vi "dfd_Check Project in Memory.vi"(8 "error in (no error)":errorcluster, 9 "filter name":string, 10 "dest path":path) -> (0 "error out":errorcluster, 1 "filter name out":string, 2 "dup dest path":path)   [LabVIEW 2017, in "NI_DigFilterLicensed.lvlib"]
uses:
  <vilib>/addons/Digital Filter Design/NI_DigFilterLicensed.lvlib
  <vilib>/addons/Digital Filter Design/_Misc.llb/dfd_Error Handlers (Single).vi
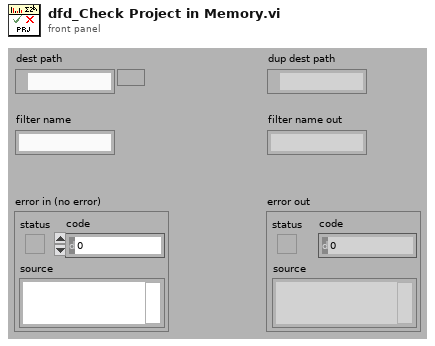
[diagram p1: front panel]
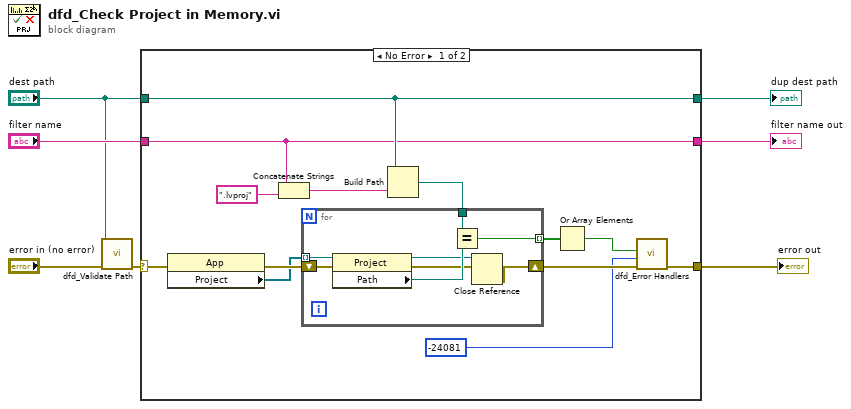
[diagram p0: block diagram]
diagram:
  n1 = call <vilib>:"dfd_Validate Path.vi"("error in (no error)"="error in (no error)", "path in"="dest path") -> ("error out"=w2:errorcluster)  [unwired: 9 out]
  n2 = case shown="No Error" w2 {
    selector: w2 -> [w18 w29]
    tunnel: "filter name" -> [w8 _]
    tunnel: "dest path" -> [w19 w30]
    tunnel: [w19 w30] -> w6
    tunnel: [w8 _] -> w5
    tunnel: [w9 w29] -> w4
    frame No Error {
      n3 = property class="App"(error in=w18) -> (error out=w13:errorcluster, "Project"=w12:refnum<vi>[])  [unwired: 1 in, 1 out]
      n4 = Concatenate Strings(w8, ".lvproj" ("string")) -> (w16:string)
      n5 = Build Path(base path=w19, name or relative path=w16) -> (appended path=w17:path)
      n6 = for {
        tunnel: w12 -> [w28] mode=indexing
        shift-right: [w21] -> w14
        shift-left: w13 -> [w27]
        tunnel: w17 -> [w25]
        tunnel: [w24] -> w15 mode=indexing
        n7 = property class="Project"(reference=w28, error in=w27) -> (reference out=w23:refnum<vi>, error out=w22:errorcluster, "Path"=w26:path)
        n8 = Equal?(x=w25, y=w26) -> (x = y?=w24:bool)
        n9 = Close Reference(reference=w23, error in (no error)=w22) -> (error out=w21:errorcluster)
      }
      n10 = Or Array Elements(Boolean array=w15) -> (logical OR=w11:bool)
      n11 = call-poly <vilib>:"dfd_Error Handlers.vi"("error in (no error)"=w14, "error code"=-24081 ("ERR_PRJ_IN_MEM"), "condition failed?"=w11) -> ("error out"=w9:errorcluster)  [unwired: 8 out]
    }
    frame Error {
    }
  }
  "error out" <- w4
  "filter name out" <- w5
  "dup dest path" <- w6
